vi "Date Stamp.vi"(5 "Time":timestamp, 6 "Format (12 Digit YmdHMS)":string="%y%m%d%H%M%S") -> (1 "U64 Out":u64, 2 "String Out":string)   [LabVIEW 2020]
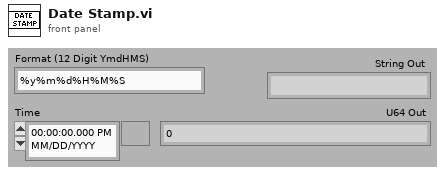
[diagram p1: front panel]
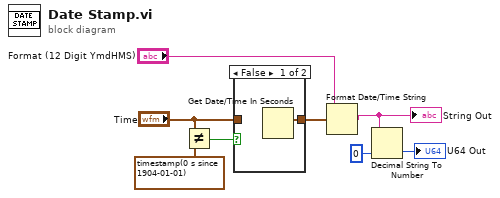
[diagram p0: block diagram]
diagram:
  n1 = Not Equal?(x="Time", y=timestamp(0 s since 1904-01-01) ("time")) -> (x != y?=w3:bool)
  n2 = case shown="False" w3 {
    tunnel: [w9 w10] -> w7
    tunnel: "Time" -> [_ w10]
    frame False {
      n3 = Get Date/Time In Seconds() -> (seconds since 1Jan1904=w9:timestamp)
    }
    frame True {
    }
  }
  n4 = Format Date/Time String(time format string (%c)="Format (12 Digit YmdHMS)", seconds (now)=w7) -> (date/time string=w1:string)  [unwired: 1 in]
  "String Out" <- w1
  n5 = Decimal String To Number(string=w1, default (0L)=u64 0 ("default (0 I32)")) -> (number=→"U64 Out":u64)  [unwired: 1 in, 1 out]
